vi "Get Consumer Values.vi"(8 "error in":errorcluster, 11 "Climate Chamber Cluster.lvclass in":refnum<class "Climate Chamber Cluster.lvclass">) -> (0 "error out":errorcluster, 1 "Consumer Ch":T1[](array[typedef]), 2 "Consumer Control":T2, 3 "Climate Chamber Cluster.lvclass out":refnum<class "Climate Chamber Cluster.lvclass">)   [LabVIEW 2023, in "Climate Chamber Cluster.lvclass"]
uses:
  Climate Chamber Cluster.lvclass
  Consumer Control.ctl
  Consumer Ch.ctl
  Climate Chamber Cluster.lvclass/Climate Chamber Cluster.ctl
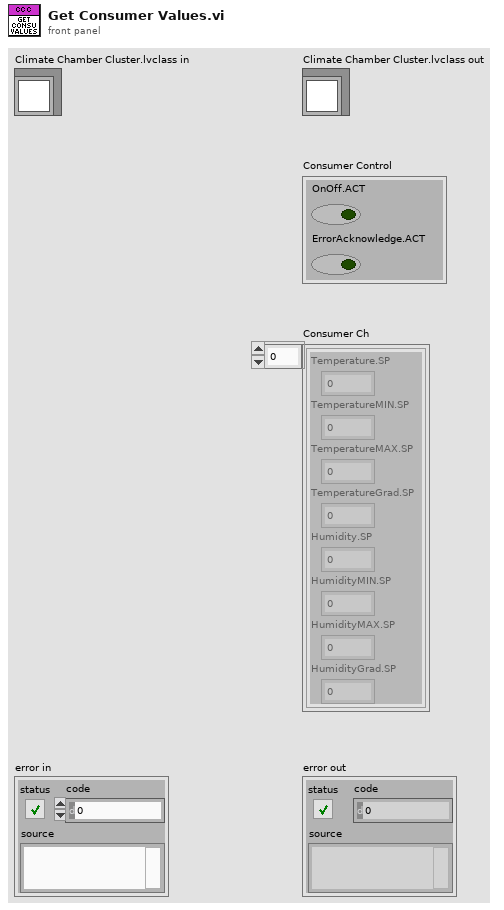
[diagram p1: front panel]
types:
  T1 = typedef "Climate Chamber Cluster.lvclass/Consumer Ch.ctl" = cluster{"Temperature.SP":dbl, "TemperatureMIN.SP":dbl, "TemperatureMAX.SP":dbl, "TemperatureGrad.SP":dbl, "Humidity.SP":dbl, "HumidityMIN.SP":dbl, "HumidityMAX.SP":dbl, "HumidityGrad.SP":dbl}
  T2 = typedef "Climate Chamber Cluster.lvclass/Consumer Control.ctl" = cluster{"OnOff.ACT":bool, "ErrorAcknowledge.ACT":bool}
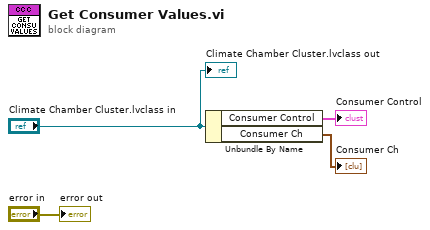
[diagram p0: block diagram]
diagram:
  n1 = Unbundle By Name("Climate Chamber Cluster.lvclass in") -> ("Consumer Control"=→"Consumer Control":T2, "Consumer Ch"=→"Consumer Ch":T1[])
  "Climate Chamber Cluster.lvclass out" <- "Climate Chamber Cluster.lvclass in"
  "error out" <- "error in"
